vi "Check for Ini files and create_ACAF.vi"(8 "error in (no error)":errorcluster) -> (0 "error out":errorcluster)   [LabVIEW 2023]
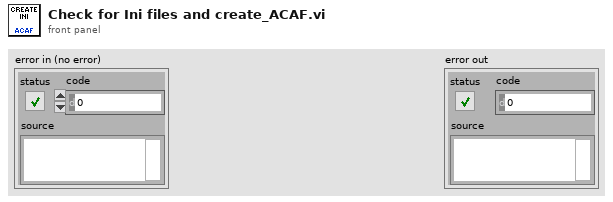
[diagram p1: front panel]
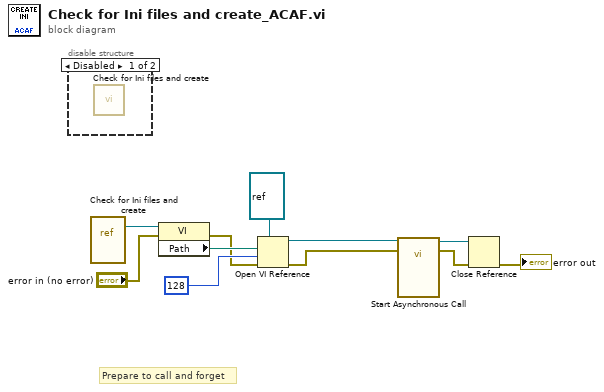
[diagram p0: block diagram]
diagram:
  # "Prepare to call and forget"
  n1 = disable-structure shown="Disabled" {
    frame Disabled {
      n2 = call "Check for Ini files and create.vi"() -> ()  [unwired: 12 in]
    }
    frame Enabled {
    }
  }
  n3 = vi-ref "Check for Ini files and create.vi"() -> (w11:refnum<vi>)
  n4 = property class="VI"(reference=w11, error in="error in (no error)") -> (error out=w1:errorcluster, "Path"=w7:path)  [unwired: 1 out]
  n5 = Open VI Reference(type specifier VI Refnum (for type only)=refnum<vi> refnum, vi path=w7, options=128, error in (no error)=w1) -> (vi reference=w2:refnum<vi>, error out=w6:errorcluster)  [unwired: 2 in]
  n6 = call-by-ref "Start Asynchronous Call"(reference=w2, error in=w6) -> (reference out=w5:refnum<vi>, error out=w4:errorcluster)  [unwired: 12 in]
  n7 = Close Reference(reference=w5, error in (no error)=w4) -> (error out=→"error out":errorcluster)
